vi "isEmpty.vi"(8 "error in (no error)":errorcluster, 11 "IComponent in":refnum<class "IComponent.lvclass">) -> (0 "error out":errorcluster, 2 "Empty?":bool, 3 "IComponent out":refnum<class "IComponent.lvclass">)   [LabVIEW 2022 SP3, in "openDAQ.lvlib" / "IBaseObject.lvlib" / "IPropertyObject.lvlib" / "IComponent.lvlib" / "IFolder.lvlib" / "IFolder.lvclass"]
uses:
  <instrlib>/openDAQ/Public/Classes/IFolder/IFolder.lvclass
  <instrlib>/openDAQ/Public/Classes/IFolder/IFolder.lvclass/IFolder.ctl
  <instrlib>/openDAQ/Public/Classes/IComponent/IComponent.lvclass
  <instrlib>/openDAQ/Binaries/Windows/x86/copendaq32.dll
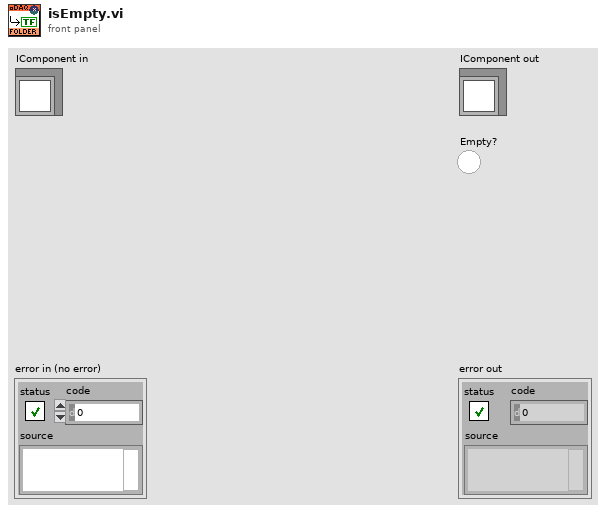
[diagram p1: front panel]
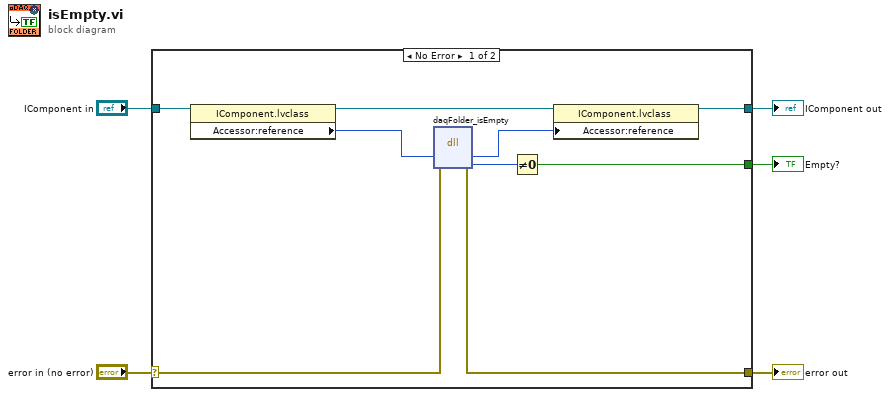
[diagram p0: block diagram]
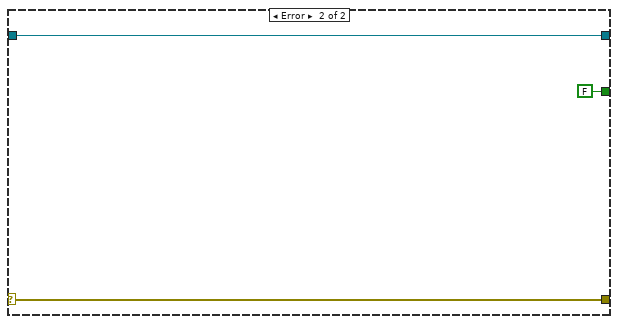
[diagram p2: hidden frame]
diagram:
  n1 = case shown="No Error" "error in (no error)" {
    selector: "error in (no error)" -> [w6 w17]
    tunnel: [w7 w17] -> w4
    tunnel: [w12 w16] -> w2
    tunnel: "IComponent in" -> [w14 w16]
    tunnel: [w8 FALSE] -> w1
    frame No Error {
      n2 = property class="IComponent.lvclass"(reference=w14) -> (reference out=w13:refnum<class "IComponent.lvclass">, "Accessor:reference"=w11:i64)  [unwired: 1 in, 1 out]
      n3 = dll-call lib="C:/Program Files (x86)/National Instruments/LabVIEW 2022/instr.lib/openDAQ/Binaries/Windows/x86/copendaq*.*" fn="daqFolder_isEmpty"(error in=w6, "folder"=w11) -> (error out=w7:errorcluster, "folder"=w10:i64, "empty"=w9:i64)  [unwired: 4 in, 1 out]
      n4 = Not Equal To 0?(x=w9) -> (x != 0?=w8:bool)
      n5 = property class="IComponent.lvclass"(reference=w13, "Accessor:reference"=w10) -> (reference out=w12:refnum<class "IComponent.lvclass">)  [unwired: 1 in, 1 out]
    }
    frame Error {
    }
  }
  "error out" <- w4
  "IComponent out" <- w2
  "Empty?" <- w1
